vi "Reset Errno Value for Calling Thread.vi"(8 "error in (no error)":errorcluster) -> (0 "error out":errorcluster, 3 "new value":T1)   [LabVIEW 2013, in "Linux Errno.lvlib"]
doc: "This VI resets the value of the errno variable for the calling thread to zero. Since errno is only set by a function when an error occurs, and not when an error does not occur, the errno variable can maintain a value from a previous function even when the error was acknowldged and handled by the application. By resetting the errno variable to zero, you can be sure that a subsequent function that sets errno was actually the source of the error."
uses:
  Linux Errno.lvlib
  Controls/Public/errno.ctl
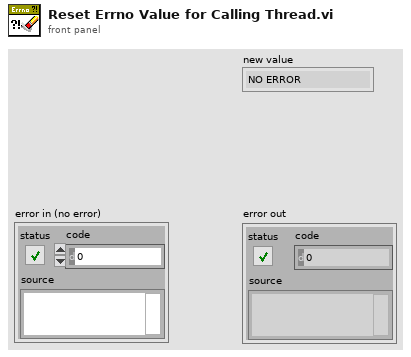
[diagram p1: front panel]
types:
  T1 = typedef "Linux Errno.lvlib/errno.ctl" = enum16{"NO ERROR", "EPERM", "ENOENT", "ESRCH", "EINTR", "EIO", "ENXIO", "E2BIG", "ENOEXEC", "EBADF", "ECHILD", "EAGAIN", "ENOMEM", "EACCES", "EFAULT", "ENOTBLK", "EBUSY", "EEXIST", "EXDEV", "ENODEV", "ENOTDIR", "EISDIR", "EINVAL", "ENFILE", "EMFILE", "ENOTTY", "ETXTBSY", "EFBIG", "ENOSPC", "ESPIPE", "EROFS", "EMLINK", "EPIPE", "EDOM", "ERANGE", "EDADLK", "ENAMETOOLONG", "ENOLCK", "ENOSYS", "ENOTEMPTY", "ELOOP", "EWOULDBLOCK", "ENOMSG", "EIDRM", "ECHRNG", "EL2NSYNC", "EL3HLT", "EL3RST", "ELNRNG", "EUNATCH", "ENOCSI", "EL2HLT", "EBADE", "EBADR", "EXFULL", "ENOANO", "EBADRQC", "EBADSLT", "EDEADLOCK", "EBFONT", "ENOSTR", "ENODATA", "ETIME", "ENOSR", "ENONET", "ENOPKG", "EREMOTE", "ENOLINK", "EADV", "ESRMNT", "ECOMM", "EPROTO", "EMULTIHOP", "EDOTDOT", "EBADMSG", "EOVERFLOW", "ENOTUNIQ", "EBADFD", "EREMCHG", "ELIBACC", "ELIBBAD", "ELIBSCN", "ELIBMAX", "ELIBEXEC", "ELISEQ", "ERESTART", "ESTRPIPE", "EUSERS", "ENOTSOCK", "EDESTADDRREQ", "EMSGSIZE", "EPROTOTYPE", "ENOPROTOOPT", "EPROTONOSUPPORT", "ESOCKTNOSUPPORT", "EOPNOTSUPP", "EPFNOSUPPORT", "EAFNOSUPPORT", "EADDRINUSE", "EADDRNOTAVAIL", "ENETDOWN", "ENETUNREACH", "ENETRESET", "ECONNABORTED", "ECONNRESET", "ENOBUFS", "EISCONN", "ENOTCONN", "ESHUTDOWN", "ETOOMANYREFS", "ETIMEDOUT", "ECONNREFUSED", "EHOSTDOWN", "EHOSTUNREACH", "EALREADY", "EINPROGRESS", "ESTALE", "EUCLEAN", "ENOTNAM", "ENAVAIL", "EISNAM", "EREMOTEIO", "EDQUOT", "ENOMEDIUM", "EMEDIUMTYPE", "ECANCELED", "ENOKEY", "EKEYEXPIRED", "EKEYREVOKED", "EKEYREJECTED", "EOWNERDEAD", "ENOTRECOVERABLE", "ERFKILL", "EHWPOISON", "UNDEFINED"}
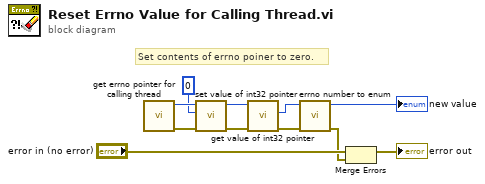
[diagram p0: block diagram]
diagram:
  # "Set contents of errno poiner to zero."
  n1 = call "get errno pointer for calling thread.vi"() -> ("error out"=w11:errorcluster, "errno pointer"=w10:u64)  [unwired: 10 in]
  n2 = call "set value of int32 pointer.vi"("error in (no error)"=w11, "value (0)"=0, "pointer in"=w10) -> ("error out"=w9:errorcluster, "pointer out"=w8:u64)  [unwired: 7 in]
  n3 = call "get value of int32 pointer.vi"("error in (no error)"=w9, "pointer in"=w8) -> ("error out"=w6:errorcluster, "value"=w5:i32)  [unwired: 7 in, 1 out]
  n4 = call "errno number to enum.vi"("error in (no error)"=w6, "errno number"=w5) -> ("error out"=w2:errorcluster, "errno enum"=→"new value":T1)  [unwired: 8 in]
  n5 = Merge Errors("error in (no error)", w2) -> (→"error out":errorcluster)
